vi "test VerifyStatic (Global).vi"(8 "error in (no error)":errorcluster, 11 "TestCase in":refnum<class "Test Numeric Test Object.lvclass">) -> (0 "error out":errorcluster, 3 "TestCase out":refnum<class "Test Numeric Test Object.lvclass">)   [LabVIEW 2009, in "Test Numeric Test Object.lvclass"]
uses:
  Test Numeric Test Object.lvclass
  Test Numeric Test Object.lvclass/Test Numeric Test Object.ctl
  Numeric Test Object/Numeric Test Object.lvclass
  <vilib>/addons/_JKI Toolkits/VI Tester/TestCase.llb/TestCase.lvclass
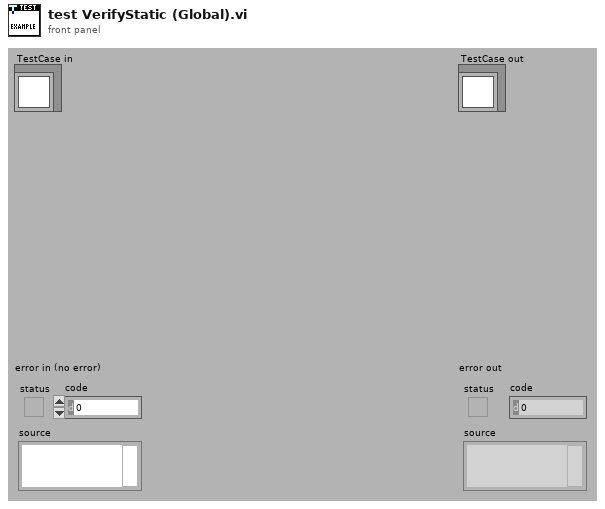
[diagram p1: front panel]
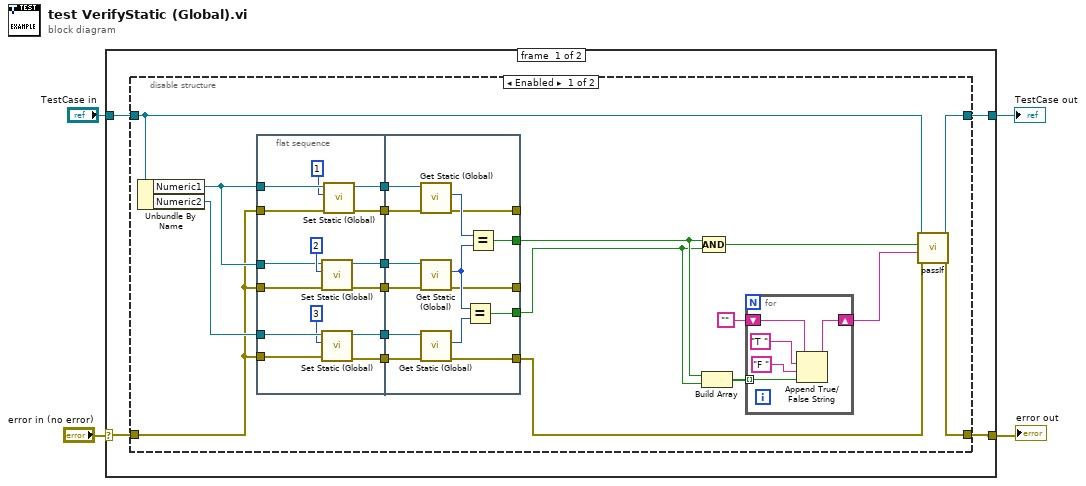
[diagram p0: block diagram]
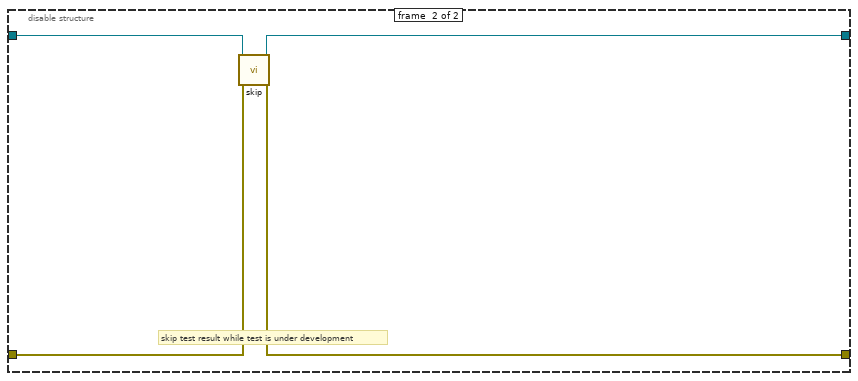
[diagram p2: hidden frame]
diagram:
  n1 = case shown="No Error" "error in (no error)" {
    selector: "error in (no error)" -> [w7 w67]
    tunnel: [w6 w67] -> w3
    tunnel: [w5 w66] -> w1
    tunnel: "TestCase in" -> [w8 w66]
    frame #0 {
      n2 = disable-structure shown="Enabled" {
        disable-tunnel: w8 -> [w25 w65]
        disable-tunnel: [w27 w62] -> w5
        disable-tunnel: w7 -> [w18 w64]
        disable-tunnel: [w26 w63] -> w6
        frame #0 {
          n3 = Unbundle By Name(w25) -> ("Numeric1"=w19:refnum<class "Numeric Test Object.lvclass">, "Numeric2"=w24:refnum<class "Numeric Test Object.lvclass">)
          n4 = flat-sequence {
            tunnel: w24 -> [w41]
            tunnel: w19 -> [w38]
            tunnel: w18 -> [w36]
            tunnel: w19 -> [w34]
            tunnel: w18 -> [w33]
            tunnel: w18 -> [w32]
            tunnel: [w42] -> w17
            tunnel: [w40] -> w16
            tunnel: [w31] -> w15
            tunnel: [w30] -> w14
            tunnel: [w29] -> w13
            tunnel: [w28] -> w12
            tunnel: w17 -> [w56]
            tunnel: w16 -> [w55]
            tunnel: w15 -> [w54]
            tunnel: w14 -> [w53]
            tunnel: w13 -> [w52]
            tunnel: w12 -> [w51]
            tunnel: [w47] -> _
            tunnel: [w46] -> _
            tunnel: [w45] -> w10
            tunnel: [w44] -> w9
            tunnel: [w43] -> w11
            frame #0 {
              n5 = call-dynamic "Set Static (Global).vi"("error in (no error)"=w33, "Int"=2, "Numeric in"=w34) -> ("error out"=w30:errorcluster, "Numeric out"=w31:refnum<class "Numeric Test Object.lvclass">)  [unwired: 7 in]
              n6 = call-dynamic "Set Static (Global).vi"("error in (no error)"=w36, "Int"=3, "Numeric in"=w41) -> ("error out"=w28:errorcluster, "Numeric out"=w29:refnum<class "Numeric Test Object.lvclass">)  [unwired: 7 in]
              n7 = call-dynamic "Set Static (Global).vi"("error in (no error)"=w32, "Int"=1, "Numeric in"=w38) -> ("error out"=w40:errorcluster, "Numeric out"=w42:refnum<class "Numeric Test Object.lvclass">)  [unwired: 7 in]
            }
            frame #1 {
              n8 = call-dynamic "Get Static (Global).vi"("error in (no error)"=w55, "Numeric in"=w56) -> ("error out"=w47:errorcluster, "Int"=w50:i32)  [unwired: 7 in, 1 out]
              n9 = call-dynamic "Get Static (Global).vi"("error in (no error)"=w53, "Numeric in"=w54) -> ("error out"=w46:errorcluster, "Int"=w49:i32)  [unwired: 7 in, 1 out]
              n10 = call-dynamic "Get Static (Global).vi"("error in (no error)"=w51, "Numeric in"=w52) -> ("error out"=w45:errorcluster, "Int"=w48:i32)  [unwired: 7 in, 1 out]
              n11 = Equal?(x=w49, y=w48) -> (x = y?=w44:bool)
              n12 = Equal?(x=w50, y=w49) -> (x = y?=w43:bool)
            }
          }
          n13 = Build Array(w11, w9) -> (w22:bool[])
          n14 = Compound Arithmetic op=AND(w11, w9) -> (w23:bool)
          n15 = for {
            tunnel: w22 -> [w61] mode=indexing
            shift-right: [w60] -> w20
            shift-left: "" -> [w57]
            n16 = Append True/False String(1:w61, 2:"F " ("false string"), 3:"T " ("true string"), 4:w57) -> (0:w60:string)
          }
          n17 = call-dynamic "passIf.vi"("error in (no error)"=w10, "message (\"\")"=w20, "pass"=w23, "TestCase in"=w25) -> ("error out"=w26:errorcluster, "TestCase out"=w27:refnum<class "Test Numeric Test Object.lvclass">)  [unwired: 6 in]
        }
        frame #1 {
          # "skip test result while test is under development"
          n18 = call <vilib>:"skip.vi"("error in (no error)"=w64, "TestCase in"=w65) -> ("error out"=w63:errorcluster, "TestCase out"=w62:refnum<class "Test Numeric Test Object.lvclass">)  [unwired: 8 in]
        }
      }
    }
    frame #1 {
    }
  }
  "error out" <- w3
  "TestCase out" <- w1
